vi "Tree.vi"   [LabVIEW 2016, in "Instrument.Cryostat.lvclass"]
uses:
  Instrument.Cryostat.lvclass
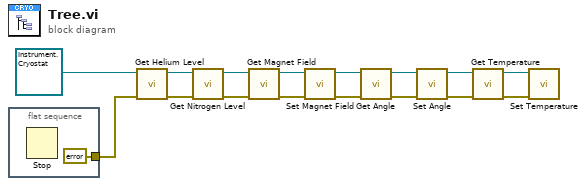
[diagram p0: block diagram]
diagram:
  n1 = flat-sequence {
    tunnel: [errorcluster {"status"=FALSE, "code"=0, "source"=""} ("error in (no error)")] -> w3
    frame #0 {
      n2 = Stop() -> ()  [unwired: 1 in]
    }
  }
  n3 = call-dynamic "Get Helium Level.vi"("error in (no error)"=w3, "Instrument.Cryostat in"=refnum<class "Instrument.Cryostat.lvclass"> refnum) -> ("error out"=w15:errorcluster, "Instrument.Cryostat out"=w16:refnum<class "Instrument.Cryostat.lvclass">)  [unwired: 7 in, 1 out]
  n4 = call-dynamic "Get Nitrogen Level.vi"("error in (no error)"=w15, "Instrument.Cryostat in"=w16) -> ("error out"=w1:errorcluster, "Instrument.Cryostat out"=w2:refnum<class "Instrument.Cryostat.lvclass">)  [unwired: 7 in, 1 out]
  n5 = call-dynamic "Get Magnet Field.vi"("error in (no error)"=w1, "Instrument.Cryostat in"=w2) -> ("error out"=w13:errorcluster, "Instrument.Cryostat out"=w14:refnum<class "Instrument.Cryostat.lvclass">)  [unwired: 6 in, 2 out]
  n6 = call-dynamic "Set Magnet Field.vi"("error in (no error)"=w13, "Instrument.Cryostat in"=w14) -> ("error out"=w11:errorcluster, "Instrument.Cryostat out"=w12:refnum<class "Instrument.Cryostat.lvclass">)  [unwired: 8 in]
  n7 = call-dynamic "Get Angle.vi"("error in (no error)"=w11, "Instrument.Cryostat in"=w12) -> ("error out"=w9:errorcluster, "Instrument.Cryostat out"=w10:refnum<class "Instrument.Cryostat.lvclass">)  [unwired: 6 in, 2 out]
  n8 = call-dynamic "Set Angle.vi"("error in (no error)"=w9, "Instrument.Cryostat in"=w10) -> ("error out"=w7:errorcluster, "Instrument.Cryostat out"=w8:refnum<class "Instrument.Cryostat.lvclass">)  [unwired: 8 in]
  n9 = call-dynamic "Get Temperature.vi"("error in (no error)"=w7, "Instrument.Cryostat in"=w8) -> ("error out"=w5:errorcluster, "Instrument.Cryostat out"=w6:refnum<class "Instrument.Cryostat.lvclass">)  [unwired: 6 in, 2 out]
  n10 = call-dynamic "Set Temperature.vi"("error in (no error)"=w5, "Instrument.Cryostat in"=w6) -> ()  [unwired: 8 in, 2 out]
